vi "Test N4L_PSM3750_Interface API.vi"() -> ()   [LabVIEW 2025, in "N4L_PSM3750_Interface.lvlib"]
doc: "N4L_PSM3750_Interface API Tester.\n\n<b>Note:</b> This VI was modified by the <b>Validate DQMH Module</b> tool to add the 'Show Main VI Diagram on Init' functionality included in DQMH 6.1.\n\n<b>Note:</b> This VI was modified by the <b>Validate DQMH Module</b> tool to upgrade its Error Reported event frame to use an improved mechanism for displaying error information.\n\n<b>Note:</b> This VI was modified by the <b>Validate DQMH Module</b> tool to upgrade it to the DQMH 5.0 approach to only call the Stop Module.vi at the end of the tester if the module wasn't originally running when the tester started.\n\n<b>Note:</b> This VI was modified by the <b>Validate DQMH Module</b> tool to remove code to stop the main loop on error, and instead display the most recent error on the tester front panel."
uses:
  N4L_PSM3750_Interface.lvlib
  Initialise--cluster.ctl
  Generator Config--cluster.ctl
  Range Config--cluster.ctl
  <vilib>/Utility/error.llb/DialogType.ctl
  <vilib>/MGI/Panel Manager/Panel/Panel/Window/Window.lvclass
  <vilib>/MGI/Panel Manager/Panel/Panel/Window/Dialog/Dialog.lvclass
  <vilib>/MGI/Panel Manager/Panel/Panel/Subpanel/Subpanel.lvclass
  <vilib>/MGI/Panel Manager/Panel/Panel/Window/Window.vi
  <vilib>/MGI/Panel Manager/Panel/Panel/Window/Dialog/Dialog.vi
  <vilib>/MGI/Panel Manager/Panel/Panel/Subpanel/Subpanel.vi
  <vilib>/MGI/Panel Manager/Panel/Panel.lvlib
panel:
  out "last error":errorcluster
  in  "Show Main VI Diagram on Init (F)":bool
  in  "Set Trim Config":T1={"AC Trim Data (Disabled)"=0, "AC Level (1)"=1.0, "Tolerance (10)"=10.0} {"Tolerance (10)" min=0.0 max=100.0 step=0.01; "AC Level (1)" min=0.0 max=10.0 step=0.0001; "AC Trim Data (Disabled)" items=["DISABLED", "CH1", "CH2"]}
  in  "Set Trim Configuration":bool
  in  "Range":T2={"Input Ranging Mode (Auto)"=enum."AUTO", "Input Input Type (Internal)"=1, "Input Selection (CH1)"=enum."CH1", "Input Connection (Main) "=0, "Input Coupling (Internal)"=enum."AC+DC", "Input Shunt Value (0,02)"=0.02, "Input Voltage Scale factor (1)"=1.0} {"Input Voltage Scale factor (1)" min=0.0 max=100000.0 step=0.001; "Input Shunt Value (0,02)" min=1e-06 max=10.0 step=1e-06; "Input Connection (Main)" items=["MAIN", "SECONDARY", "DIFFERENTIAL"]; "Input Input Type (Internal)" items=["DISABLED", "INTERNAL", "EXTERNAL SHUNT"]}
  in  "Set Range":bool
  in  "Generator Output":enum16{"OFF", "ON"}(ring)
  in  "Set Generator Output":bool
  in  "Generator Configuration":T3={"Waveform"=enum."Sinewave", "Frequency (1000)"=1000.0, "Amplitude (2)"=2.0, "Offset (0)"=0.0} {"Offset (0)" min=-10.0 max=10.0 step=0.0001; "Amplitude (2)" min=0.0 max=10.0 step=1e-05; "Frequency (1000)" min=0.0 max=35000000.0 step=0.0001}
  in  "Set Generator Configuration":bool
  in  "Reset N4L Instrument":bool
  in  "Close N4L Connection":bool
  out "State Map":map{string, dbl}(c390)
  in  "N4L Initialise":T4={"VISA resource name"="COM4", "Baud Rate"=19200, "ID Query"=FALSE, "Reset"=FALSE} {"Baud Rate" items=["300"=300, "600"=600, "1200"=1200, "2400"=2400, "4800"=4800, "9600"=9600, "19200"=19200]}
  in  "Initialise N4L Connection":bool
  in  "Autoshow?":bool
  in  "Panel Type":enum16{"Window", "Dialog", "Subpanel"}(ring)
  in  "Change Panel":bool
  in  "Tab Control":enum32{"Status", "Subpanel"}(tab)
  out "Status":string
  in  "Show Block Diagram":bool
  in  "Stop Module":bool
  in  "Start Module":bool
  in  "Hide Module Panel":bool
  in  "Show Module Panel":bool
  out "Module Running?":bool
  # "This VI tests the API for the Module."
  # "Change Panel"
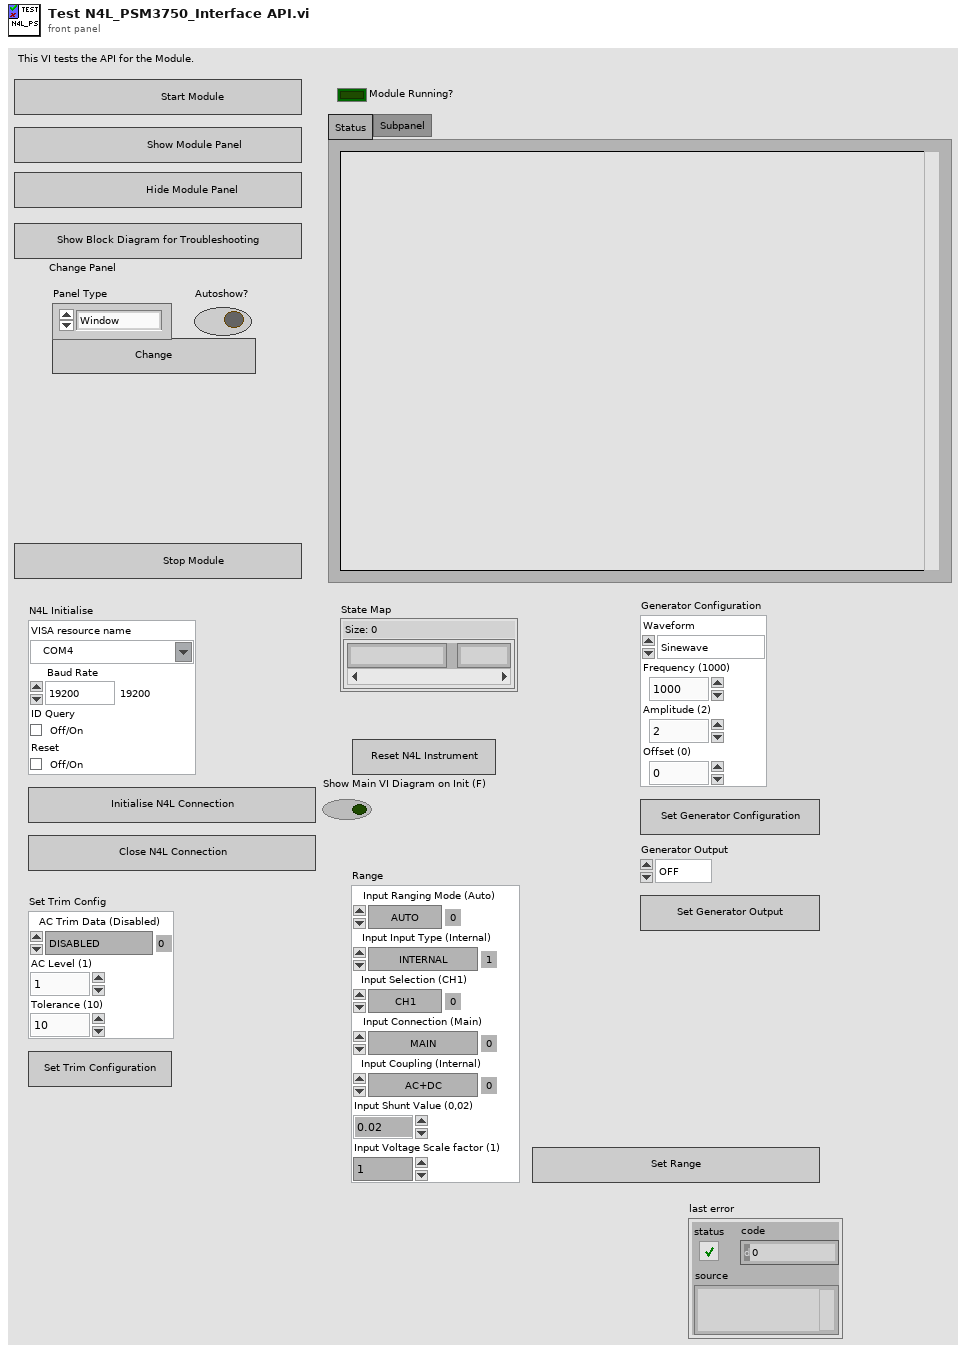
[diagram p1: front panel]
types:
  T1 = cluster{"AC Trim Data (Disabled)":u16, "AC Level (1)":dbl, "Tolerance (10)":dbl}
  T2 = typedef "N4L_PSM3750_Interface.lvlib/Range Config--cluster.ctl" = cluster{"Input Ranging Mode (Auto)":enum16{"AUTO", "UPAUTO", "1mV", "3mV", "10mV", "30mV", "100mV", "300mV", "1V", "3V", "10V"}, "Input Input Type (Internal)":u16, "Input Selection (CH1)":enum16{"CH1", "CH2"}, "Input Connection (Main) ":u16, "Input Coupling (Internal)":enum16{"AC+DC", "AC"}, "Input Shunt Value (0,02)":dbl, "Input Voltage Scale factor (1)":dbl}
  T3 = typedef "N4L_PSM3750_Interface.lvlib/Generator Config--cluster.ctl" = cluster{"Waveform":enum16{"Sinewave", "Square"}, "Frequency (1000)":dbl, "Amplitude (2)":dbl, "Offset (0)":dbl}
  T4 = typedef "N4L_PSM3750_Interface.lvlib/Initialise--cluster.ctl" = cluster{"VISA resource name":refnum<visa-resource-name>, "Baud Rate":u32, "ID Query":bool, "Reset":bool}
  T5 = typedef "N4L_PSM3750_Interface.lvlib/Broadcast Events--cluster.ctl" = cluster{"Module Did Init":refnum<user-event>, "Status Updated":refnum<user-event>, "Error Reported":refnum<user-event>, "Module Did Stop":refnum<user-event>, "Update Module Execution Status":refnum<user-event>, "Broadcast State":refnum<user-event>}
  T6 = typedef "DialogType.ctl" = u16
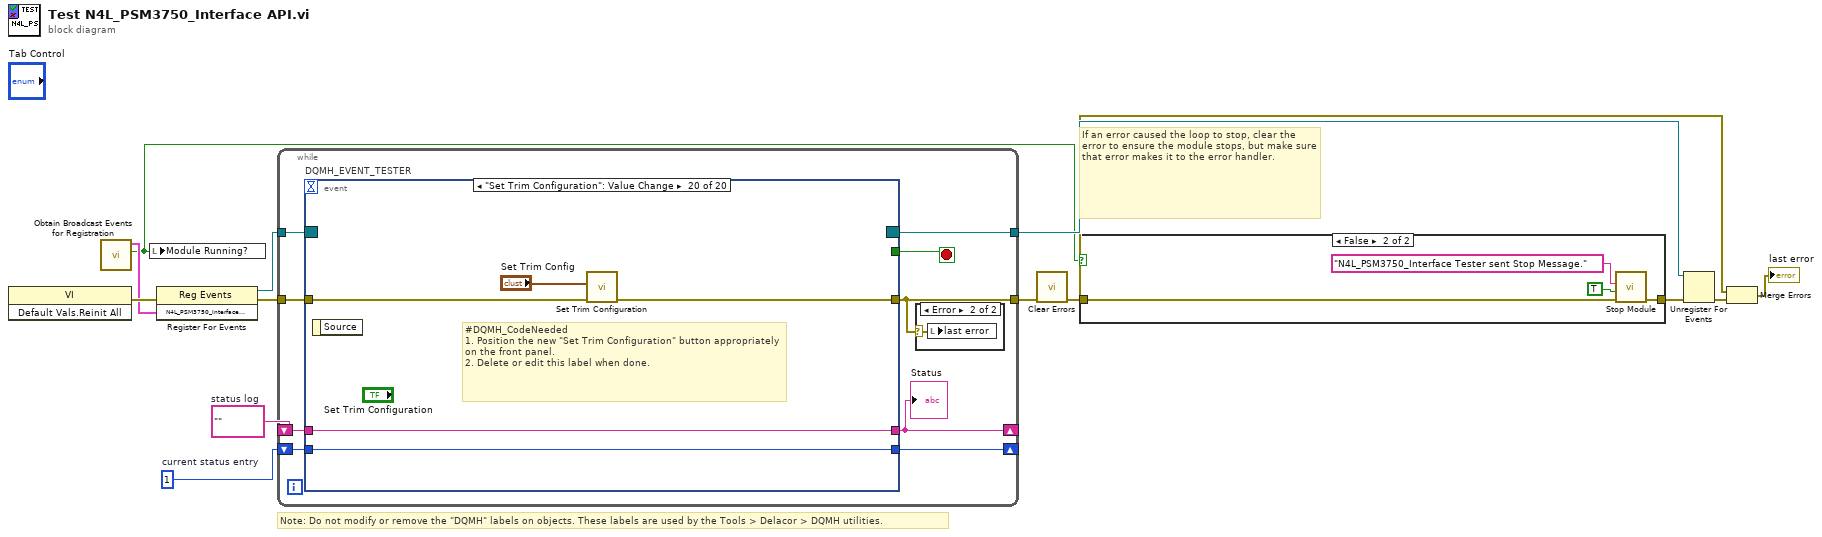
[diagram p0: block diagram]
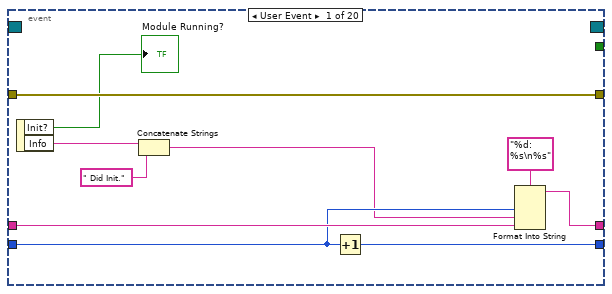
[diagram p4: hidden frame]
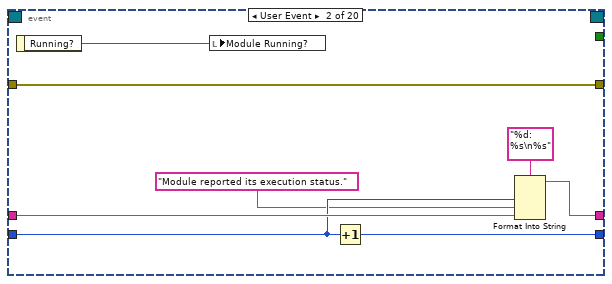
[diagram p5: hidden frame]
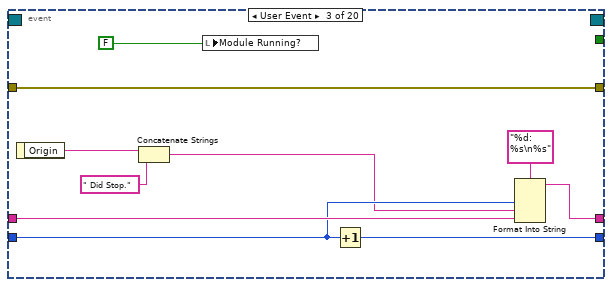
[diagram p6: hidden frame]
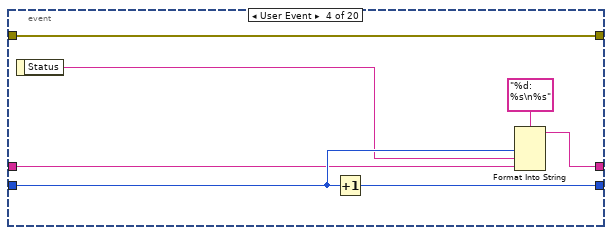
[diagram p7: hidden frame]
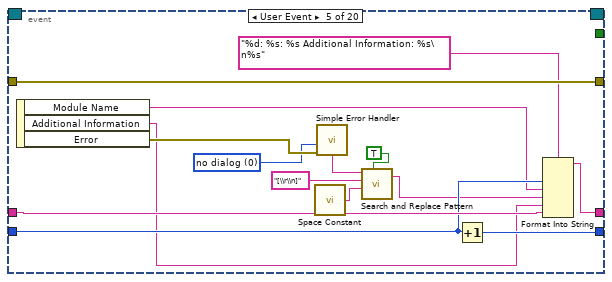
[diagram p8: hidden frame]
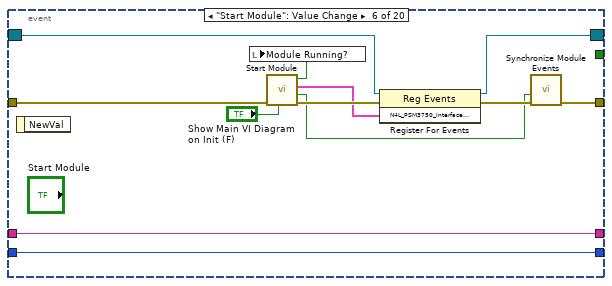
[diagram p9: hidden frame]
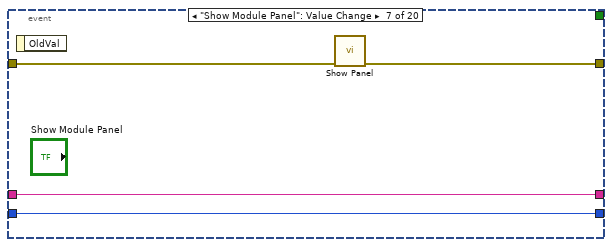
[diagram p10: hidden frame]
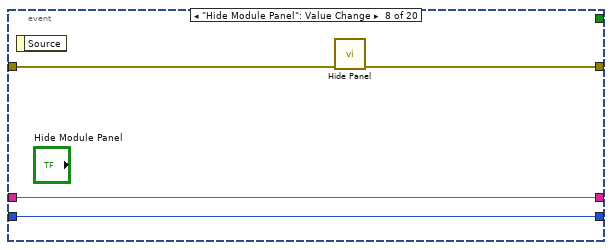
[diagram p11: hidden frame]
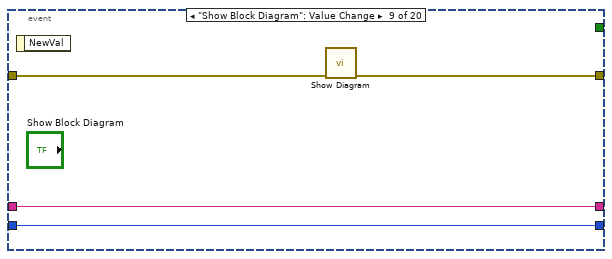
[diagram p12: hidden frame]
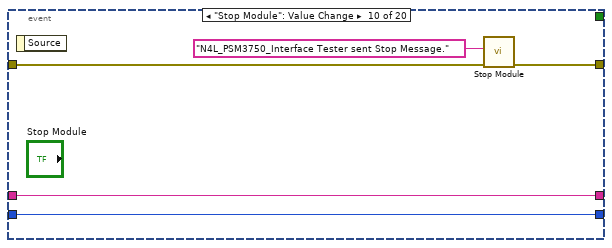
[diagram p13: hidden frame]
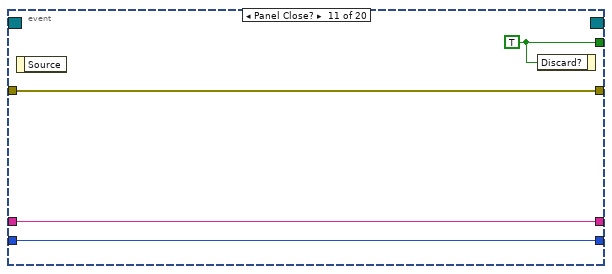
[diagram p14: hidden frame]
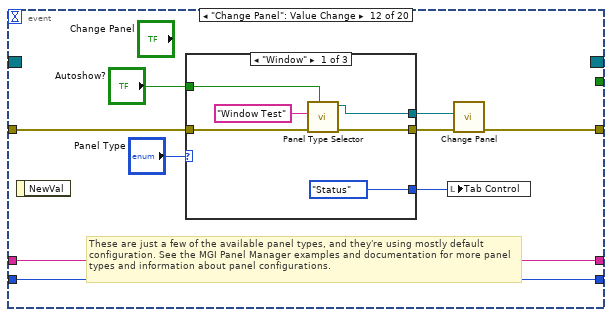
[diagram p15: hidden frame]
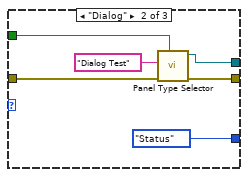
[diagram p16: hidden frame]
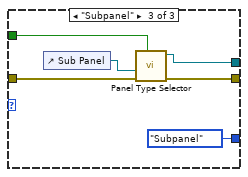
[diagram p17: hidden frame]
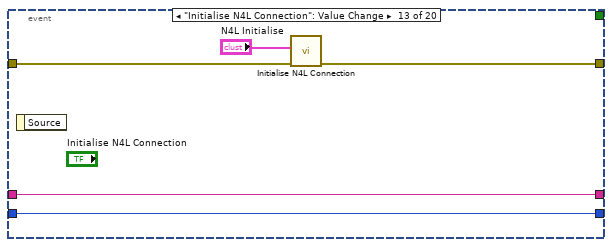
[diagram p18: hidden frame]
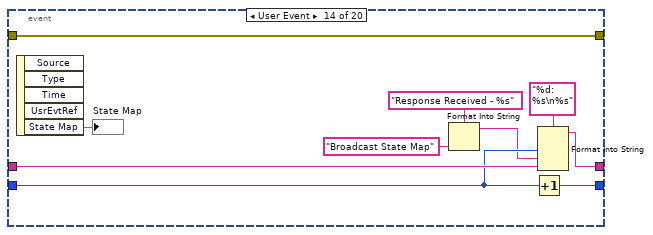
[diagram p19: hidden frame]
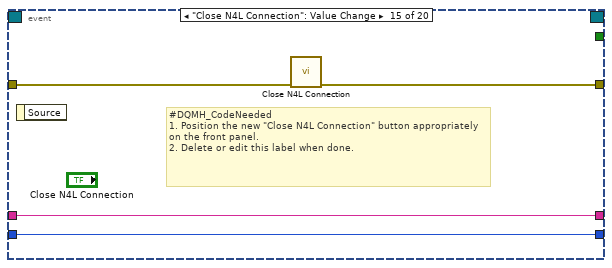
[diagram p20: hidden frame]
diagram:
  w10 = 1  # current status entry
  w11 = ""  # status log
  # "If an error caused the loop to stop, clear the error to ensure the module stops, but make sure that error makes it to the error handler."
  # "Note: Do not modify or remove the \"DQMH\" labels on objects. These labels are used by the Tools > Delacor > DQMH utilities."
  n1 = invoke class="VI" method="Default Vals.Reinit All"() -> (error out=w9:errorcluster)  [unwired: 3 in, 2 out]
  n2 = call "Obtain Broadcast Events for Registration.vi"() -> ("Already running?"=w2:bool, "N4L_PSM3750_Interface Broadcast Events"=w7:T5)  [unwired: 9 in, 1 out]
  n3 = local write "Module Running?"(w2) -> ()
  n4 = register-events(error in=w9, w7) -> (reference out=w6:refnum<event-registration>, error out=w8:errorcluster)  [unwired: 1 in]
  n5 = while {
    tunnel: w6 -> [w22]
    tunnel: [w15] -> w3
    shift-right: [w18] -> _
    shift-left: w11 -> [w20]
    shift-right: [w19] -> _
    shift-left: w10 -> [w21]
    tunnel: w8 -> [w17]
    tunnel: [w16] -> w5
    stop <- w14 stop-if-true
    n6 = event "DQMH_EVENT_TESTER" shown="[19] \"Set Trim Configuration\": Value Change" {
      selector: w22 -> [_ _ _ _ _ w79 _ _ _ _ _ _ _ _ _ _ _ _ _ _]
      dyn-events: [_ _ _ _ _ w78 _ _ _ _ _ _ _ _ _ _ _ _ _ _] -> w16
      timeout: _ -> [_ _ _ _ _ _ _ _ _ _ _ _ _ _ _ _ _ _ _ _]
      tunnel: [_ _ _ _ _ _ _ _ _ _ w106 _ _ _ _ _ _ _ _ _] -> w14
      tunnel: [w33 w35 w42 w52 w73 w77 w89 w93 w94 w100 w103 w113 w135 w148 w149 w153 w158 w163 w168 w173] -> w15
      tunnel: w21 -> [w29 w39 w49 w55 w70 w82 w87 w91 w95 w101 w104 w114 w136 w145 w150 w154 w159 w164 w169 w174]
      tunnel: w20 -> [w30 w40 w50 w54 w72 w83 w88 w92 w96 w102 w105 w115 w137 w147 w151 w155 w160 w165 w170 w175]
      tunnel: [w27 w37 w47 w56 w71 w83 w88 w92 w96 w102 w105 w115 w137 w146 w151 w155 w160 w165 w170 w175] -> w18
      tunnel: [w28 w38 w48 w58 w69 w82 w87 w91 w95 w101 w104 w114 w136 w144 w150 w154 w159 w164 w169 w174] -> w19
      tunnel: w17 -> [w33 w35 w42 w52 w73 w75 w86 w90 w97 w98 w103 w112 w138 w148 w152 w156 w161 w166 w171 w176]
      event User Event {
        n7 = event-data() -> ("Init?"=→"Module Running?":bool, "Info"=w26:string)  [unwired: 1 in]
        n8 = Concatenate Strings(w26, " Did Init.") -> (w25:string)
        n9 = Increment(x=w29) -> (x+1=w28:i32)
        n10 = Format Into String(format string="%d: %s\n%s", w29, w25, w30) -> (resulting string=w27:string)  [unwired: 2 in, 1 out]
      }
      event User Event {
        n11 = event-data() -> ("Running?"=w34:bool)  [unwired: 1 in]
        n12 = local write "Module Running?"(w34) -> ()
        n13 = Increment(x=w39) -> (x+1=w38:i32)
        n14 = Format Into String(format string="%d: %s\n%s", w39, "Module reported its execution status.", w40) -> (resulting string=w37:string)  [unwired: 2 in, 1 out]
      }
      event User Event {
        n15 = event-data() -> ("Origin"=w46:string)  [unwired: 1 in]
        n16 = Concatenate Strings(w46, " Did Stop.") -> (w45:string)
        n17 = local write "Module Running?"(FALSE ("Module Did Init?")) -> ()
        n18 = Increment(x=w49) -> (x+1=w48:i32)
        n19 = Format Into String(format string="%d: %s\n%s", w49, w45, w50) -> (resulting string=w47:string)  [unwired: 2 in, 1 out]
      }
      event User Event {
        n20 = event-data() -> ("Status"=w53:string)  [unwired: 1 in]
        n21 = Increment(x=w55) -> (x+1=w58:i32)
        n22 = Format Into String(format string="%d: %s\n%s", w55, w53, w54) -> (resulting string=w56:string)  [unwired: 2 in, 1 out]
      }
      event User Event {
        w65 = T6 0 items=["no dialog", "OK message", "continue or stop message", "OK message + warnings", "continue/stop + warnings"] ("type of dialog (OK msg:1)")
        n23 = event-data() -> ("Module Name"=w66:string, "Additional Information"=w67:string, "Error"=w68:errorcluster)  [unwired: 1 in]
        n24 = call <vilib>:"Space Constant.vi"() -> ("String"=w61:string)
        n25 = call <vilib>:"Simple Error Handler.vi"("type of dialog (OK msg:1)"=w65, "error in (no error)"=w68) -> ("message"=w64:string)  [unwired: 3 in, 4 out]
        n26 = call <vilib>:"Search and Replace Pattern.vi"("string"=w64, "regular expression (\"\")"="[\\r\\n]" ("regular expression (\"\")"), "replace string (\"\")"=w61, "replace all? (F)"=TRUE ("replace all CR/LF with spaces")) -> ("result string"=w63:string)  [unwired: 1 in, 1 out]
        n27 = Increment(x=w70) -> (x+1=w69:i32)
        n28 = Format Into String(format string="%d: %s: %s Additional Information: %s\n%s", w70, w66, w63, w67, w72) -> (resulting string=w71:string)  [unwired: 2 in, 1 out]
      }
      event "Start Module": Value Change {
        n29 = event-data() -> ()  [unwired: 1 in, 1 out]
        n30 = call "Start Module.vi"("Show Main VI Diagram on Init (F)"="Show Main VI Diagram on Init (F)", "error in (no error)"=w75) -> ("error out"=w84:errorcluster, "Wait for Event Sync?"=w81:bool, "N4L_PSM3750_Interface Broadcast Events"=w80:T5, "Module Was Already Running?"=w76:bool)  [unwired: 5 in, 1 out]
        n31 = local write "Module Running?"(w76) -> ()
        n32 = register-events(reference=w79, error in=w84, w80) -> (reference out=w78:refnum<event-registration>, error out=w85:errorcluster)
        n33 = call "Synchronize Module Events.vi"("error in (no error)"=w85, "Wait for Event Sync?"=w81) -> ("error out"=w77:errorcluster)  [unwired: 9 in]
      }
      event "Show Module Panel": Value Change {
        n34 = event-data() -> ()  [unwired: 1 in, 1 out]
        n35 = call "Show Panel.vi"("error in (no error)"=w86) -> ("error out"=w89:errorcluster)  [unwired: 10 in]
      }
      event "Hide Module Panel": Value Change {
        n36 = event-data() -> ()  [unwired: 1 in, 1 out]
        n37 = call "Hide Panel.vi"("error in (no error)"=w90) -> ("error out"=w93:errorcluster)  [unwired: 10 in]
      }
      event "Show Block Diagram": Value Change {
        n38 = event-data() -> ()  [unwired: 1 in, 1 out]
        n39 = call "Show Diagram.vi"("error in (no error)"=w97) -> ("error out"=w94:errorcluster)  [unwired: 10 in]
      }
      event "Stop Module": Value Change {
        n40 = event-data() -> ()  [unwired: 1 in, 1 out]
        n41 = call "Stop Module.vi"("error in (no error)"=w98, "Origin"="N4L_PSM3750_Interface Tester sent Stop Message.") -> ("error out"=w100:errorcluster)  [unwired: 9 in]
      }
      event Panel Close? {
        w106 = TRUE ("Discard?")
        n42 = event-data() -> ()  [unwired: 1 in, 1 out]
        n43 = event-data("Discard?"=w106) -> ()  [unwired: 1 in, 1 out]
      }
      event "Change Panel": Value Change {
        # "These are just a few of the available panel types, and they're using mostly default configuration. See the MGI Panel Manager examples and documentation for more panel types and information about panel configurations."
        n44 = event-data() -> ()  [unwired: 1 in, 1 out]
        n45 = case shown="\"Window\"" "Panel Type" {
          tunnel: w112 -> [w121 w127 w133]
          tunnel: [w120 w126 w132] -> w111
          tunnel: [w119 w125 w131] -> w110
          tunnel: [enum32{"Status", "Subpanel"}."Status" ("Tab Control") enum32{"Status", "Subpanel"}."Status" ("Tab Control") enum32{"Status", "Subpanel"}."Subpanel" ("Tab Control")] -> w108
          tunnel: "Autoshow?" -> [w116 w122 w128]
          frame "Window" {
            n46 = call-poly <vilib>:"Panel Type Selector.vi"("Autoshow? (T)"=w116, "error in (no error)"=w121, "Default Title"="Window Test") -> ("error out"=w120:errorcluster, "Window out"=w119:refnum<class "Window.lvclass">)  [unwired: 7 in]
          }
          frame "Dialog" {
            n47 = call-poly <vilib>:"Panel Type Selector.vi"("Autoshow? (T)"=w122, "Error In"=w127, "Default Title"="Dialog Test") -> ("Error Out"=w126:errorcluster, "Dialog out"=w125:refnum<class "Dialog.lvclass">)  [unwired: 7 in]
          }
          frame "Subpanel" {
            n48 = control-ref of="Sub Panel"() -> (w130:refnum<vi>)
            n49 = call-poly <vilib>:"Panel Type Selector.vi"("Autoshow? (T)"=w128, "Error In"=w133, "Sub Panel"=w130) -> ("Error Out"=w132:errorcluster, "Subpanel Out"=w131:refnum<class "Subpanel.lvclass">)  [unwired: 7 in]
          }
        }
        n50 = local write "Tab Control"(w108) -> ()
        n51 = call "Change Panel.vi"("error in (no error)"=w111, "New Panel"=w110) -> ("error out"=w113:errorcluster)  [unwired: 9 in]
      }
      event "Initialise N4L Connection": Value Change {
        n52 = event-data() -> ()  [unwired: 1 in, 1 out]
        n53 = call "Initialise N4L Connection.vi"("error in"=w138, "N4L Initialise"="N4L Initialise") -> ("error out"=w135:errorcluster)  [unwired: 9 in]
      }
      event User Event {
        n54 = event-data() -> ("State Map"=→"State Map":map{string, dbl})  [unwired: 1 in, 4 out]
        n55 = Format Into String(format string="Response Received - %s", "Broadcast State Map" ("input 1")) -> (resulting string=w141:string)  [unwired: 2 in, 1 out]
        n56 = Increment(x=w145) -> (x+1=w144:i32)
        n57 = Format Into String(format string="%d: %s\n%s", w145, w141, w147) -> (resulting string=w146:string)  [unwired: 2 in, 1 out]
      }
      event "Close N4L Connection": Value Change {
        # "#DQMH_CodeNeeded\n1. Position the new \"Close N4L Connection\" button appropriately on the front panel.\n2. Delete or edit this label when done."
        n58 = event-data() -> ()  [unwired: 1 in, 1 out]
        n59 = call "Close N4L Connection.vi"("error in"=w152) -> ("error out"=w149:errorcluster)  [unwired: 10 in]
      }
      event "Reset N4L Instrument": Value Change {
        n60 = event-data() -> ()  [unwired: 1 in, 1 out]
        n61 = call "Reset N4L Instrument.vi"("error in"=w156) -> ("error out"=w153:errorcluster)  [unwired: 10 in]
      }
      event "Set Generator Configuration": Value Change {
        # "#DQMH_CodeNeeded\n1. Position the new \"Set Generator Configuration\" button appropriately on the front panel.\n2. Delete or edit this label when done."
        n62 = event-data() -> ()  [unwired: 1 in, 1 out]
        n63 = call "Set Generator Configuration.vi"("error in"=w161, "Generator Configuration"="Generator Configuration") -> ("error out"=w158:errorcluster)  [unwired: 9 in]
      }
      event "Set Generator Output": Value Change {
        # "#DQMH_CodeNeeded\n1. Position the new \"Set Generator Output\" button appropriately on the front panel.\n2. Delete or edit this label when done."
        n64 = event-data() -> ()  [unwired: 1 in, 1 out]
        n65 = call "Set Generator Output.vi"("error in"=w166, "Generator Output"="Generator Output") -> ("error out"=w163:errorcluster)  [unwired: 9 in]
      }
      event "Set Range": Value Change {
        # "#DQMH_CodeNeeded\n1. Position the new \"Set Range\" button appropriately on the front panel.\n2. Delete or edit this label when done."
        n66 = event-data() -> ()  [unwired: 1 in, 1 out]
        n67 = call "Set Range.vi"("error in"=w171, "Range"="Range") -> ("error out"=w168:errorcluster)  [unwired: 9 in]
      }
      event "Set Trim Configuration": Value Change {
        # "#DQMH_CodeNeeded\n1. Position the new \"Set Trim Configuration\" button appropriately on the front panel.\n2. Delete or edit this label when done."
        n68 = event-data() -> ()  [unwired: 1 in, 1 out]
        n69 = call "Set Trim Configuration.vi"("error in"=w176, "Set Trim Config"="Set Trim Config") -> ("error out"=w173:errorcluster)  [unwired: 9 in]
      }
    }
    "Status" <- w18
    n70 = case "DQMH_TESTER_ERROR_LOCAL" shown="Error" w15 {
      selector: w15 -> [_ w23]
      frame No Error {
      }
      frame Error {
        n71 = local write "last error"(w23) -> ()
      }
    }
  }
  n72 = call <vilib>:"Clear Errors.vi"("error in (no error)"=w3) -> ("error out"=w4:errorcluster)  [unwired: 5 in, 1 out]
  n73 = case shown="False" w2 {
    tunnel: [w177 w181] -> w12
    tunnel: w4 -> [w177 w178]
    frame True {
    }
    frame False {
      n74 = call "Stop Module.vi"("error in (no error)"=w178, "Wait for Module to Stop? (F)"=TRUE ("Wait for Module to stop?"), "Origin"="N4L_PSM3750_Interface Tester sent Stop Message.") -> ("error out"=w181:errorcluster)  [unwired: 8 in]
    }
  }
  n75 = Unregister For Events(event registration refnum=w5, error in=w12) -> (error out=w13:errorcluster)
  n76 = Merge Errors(w3, w13) -> (→"last error":errorcluster)
